vi "弹窗-累积超限通知.vi"(11 "报警信息":T1) -> ()   [LabVIEW 2017]
panel:
  out "累积剂量":string
  out "起始时间":string
  out "记录时间":string
  out "报警对象":string
  # "报警对象"
  # "起始时间"
  # "报警时间"
  # "累积剂量"
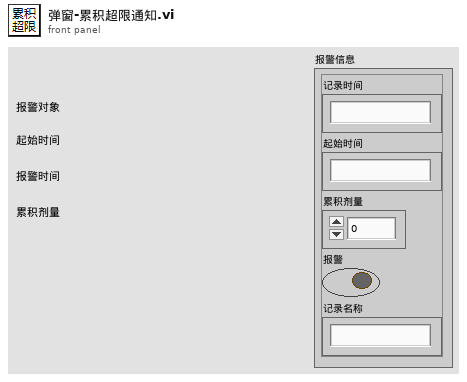
[diagram p1: front panel]
types:
  T1 = cluster{"记录时间":string, "起始时间":string, "累积剂量":dbl, "报警":bool, "记录名称":string}
  T2 = enum32{"Invalid", "Standard", "Closed", "Hidden", "Minimized", "Maximized"}
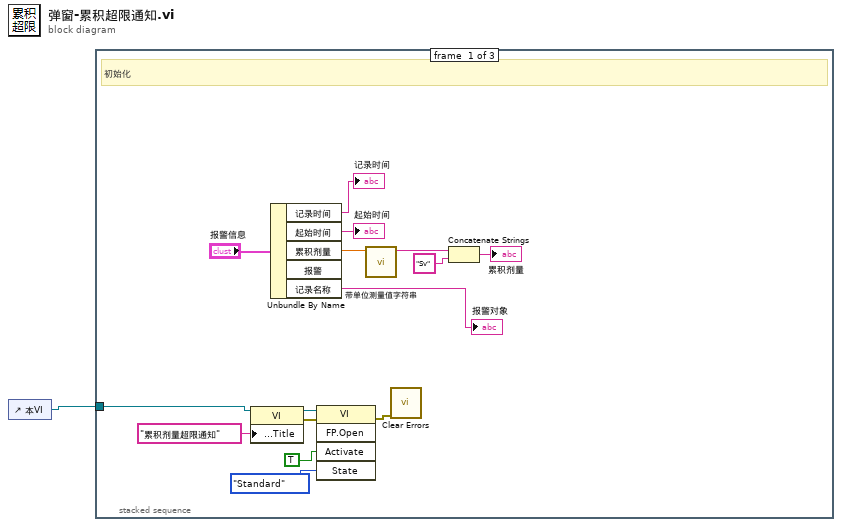
[diagram p0: block diagram]
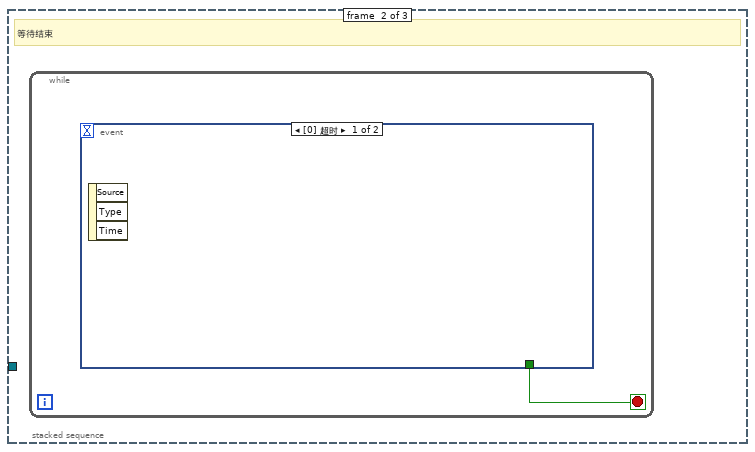
[diagram p2: hidden frame]
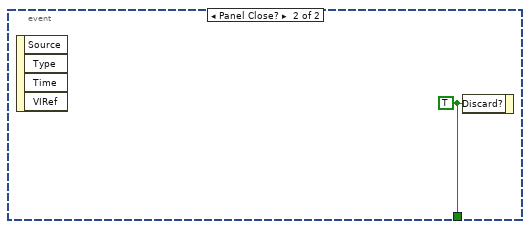
[diagram p3: hidden frame]
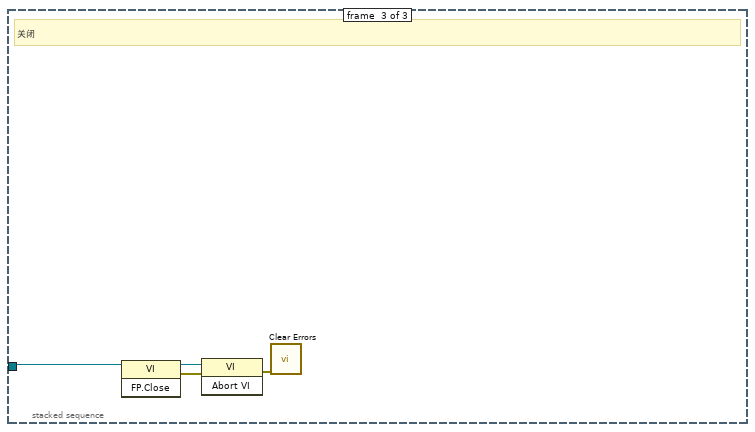
[diagram p4: hidden frame]
diagram:
  n1 = control-ref of="本VI"() -> (w1:refnum<vi>)
  n2 = stacked-sequence {
    tunnel: w1 -> [w3 _ w22]
    frame #0 {
      # "初始化"
      n3 = property class="VI"(reference=w3, "Front Panel.Title"="累积剂量超限通知" ("前面板窗口:标题")) -> (reference out=w8:refnum<vi>, error out=w7:errorcluster)  [unwired: 1 in]
      n4 = Unbundle By Name("报警信息") -> ("记录时间"=→"记录时间":string, "起始时间"=→"起始时间":string, "累积剂量"=w13:dbl, "记录名称"=→"报警对象":string)  [unwired: 1 out]
      n5 = invoke class="VI" method="FP.Open"(reference=w8, error in=w7, "Activate"=TRUE ("激活？"), "State"=T2."Standard" ("状态")) -> (error out=w4:errorcluster)  [unwired: 1 in, 4 out]
      n6 = call "带单位测量值字符串.vi"("测量值"=w13) -> ("结果"=w12:string)  [unwired: 10 in]
      n7 = call <vilib>:"Clear Errors.vi"("error in (no error)"=w4) -> ()  [unwired: 5 in, 2 out]
      n8 = Concatenate Strings(w12, "Sv" ("字符串")) -> (→"累积剂量":string)
    }
    frame #1 {
      # "等待结束"
      n9 = while {
        stop <- w17 stop-if-true
        n10 = event shown="[0] 超时" {
          selector: _ -> [_ _]
          dyn-events: _ -> [_ _]
          timeout: _ -> [_ _]
          tunnel: [_ w18] -> w17
          event Timeout {
            n11 = event-data() -> ()  [unwired: 1 in, 3 out]
          }
          event Panel Close? {
            w18 = TRUE ("放弃？")
            n12 = event-data() -> ()  [unwired: 1 in, 4 out]
            n13 = event-data("Discard?"=w18) -> ()  [unwired: 1 in, 1 out]
          }
        }
      }
    }
    frame #2 {
      # "关闭"
      n14 = invoke class="VI" method="FP.Close"(reference=w22) -> (reference out=w21:refnum<vi>, error out=w20:errorcluster)  [unwired: 2 in, 1 out]
      n15 = invoke class="VI" method="Abort VI"(reference=w21, error in=w20) -> (error out=w19:errorcluster)  [unwired: 1 in, 2 out]
      n16 = call <vilib>:"Clear Errors.vi"("error in (no error)"=w19) -> ()  [unwired: 5 in, 2 out]
    }
  }
